vi "RSZVB Set Converter Power Offset.vi"(6 "Port Power Offset (0)":dbl format="%^.3e", 7 "Offset Parameter (1)":i32(ring)=1 items=["Only", "Add Channel Power"], 8 "error in (no error)":errorcluster {"code" format="%.0x"}, 9 "Port (1)":i32=1, 10 "Channel (1)":i32=1, 11 "VISA session":refnum<visa-resource-name>) -> (0 "error out":errorcluster {"code" format="%.0x"}, 3 "dup VISA session":refnum<visa-resource-name>)   [LabVIEW 2011]
doc: "This VI defines a source power or a power offset relative to the channel power (SOURce<Ch>:POWer<Pt>[:LEVel][:IMMediate][:AMPlitude]) for a frequency converter port <Pt>. The command is available for converters with electronic attenuators (R&S ZVA-ZxxxE). An additional Cal Power Offset can be defined via SOURce<Ch>:POWer<Pt>:CORRection:LEVel:OFFSet. \n\n\nNotes:\n\n(1) This command is available for frequency converters with electronic attenuators R&S ZVA-ZxxxE.\n\nRemote-control command(s):\nSOURce<Ch>:POWer<Pt>:CONVerter:OFFSet <numeric_value>, ONLY | CPADd"
uses:
  _utility/RSZVB Global Data.vi
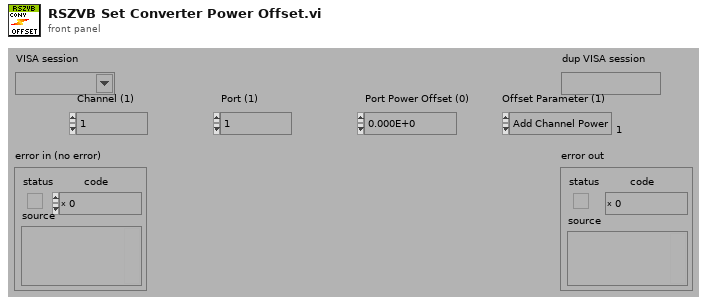
[diagram p1: front panel]
types:
  T1 = cluster{"Error Checking (T: On)":bool, "Installed Options":string[], "Data Valid?":bool, "Ports":i32, "Model":string[], "Option Checking (T: On)":bool}[]
  T2 = cluster{"Error Checking (T: On)":bool, "Installed Options":string[], "Data Valid?":bool, "Ports":i32, "Model":string[], "Option Checking (T: On)":bool}
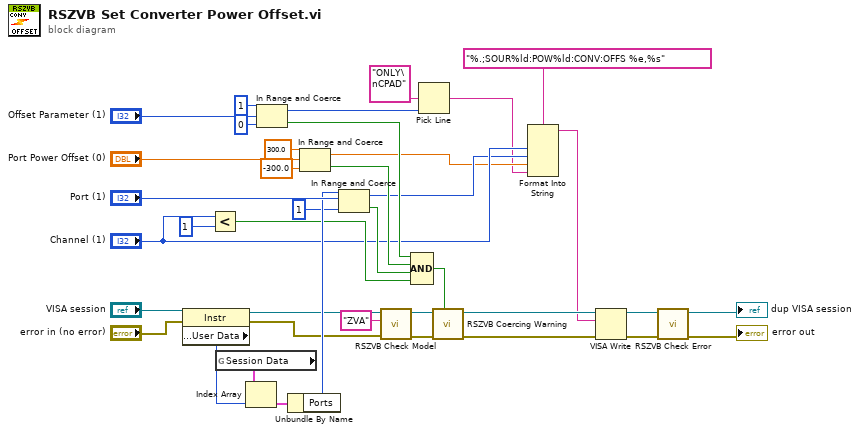
[diagram p0: block diagram]
diagram:
  n1 = property class="Instr"(reference="VISA session", error in="error in (no error)") -> (reference out=w1:refnum<visa-resource-name>, error out=w2:errorcluster, "General Settings:User Data"=w37:u32)
  n2 = Less?(x="Channel (1)", y=1) -> (x < y?=w21:bool)
  n3 = global read "RSZVB Global Data.vi" "Session Data"() -> (w38:T1)
  n4 = Index Array(array=w38, index=w37) -> (element=w39:T2)
  n5 = In Range and Coerce(upper limit=1, x="Offset Parameter (1)", lower limit=0) -> (coerced(x)=w19:i32, In Range?=w24:bool)
  n6 = Unbundle By Name(w39) -> ("Ports"=w33:i32)
  n7 = In Range and Coerce(upper limit=300.0, x="Port Power Offset (0)", lower limit=-300.0) -> (coerced(x)=w14:dbl, In Range?=w23:bool)
  n8 = In Range and Coerce(upper limit=w33, x="Port (1)", lower limit=1) -> (coerced(x)=w15:i32, In Range?=w22:bool)
  n9 = call "RSZVB Check Model.vi"("error in (no error)"=w2, "Model"="ZVA", "VISA session"=w1) -> ("error out"=w4:errorcluster, "dup VISA session"=w3:refnum<visa-resource-name>)  [unwired: 7 in]
  n10 = Compound Arithmetic op=AND(w24, w23, w22, w21) -> (w20:bool)
  n11 = Pick Line(multi-line string="ONLY\nCPAD", line index=w19) -> (output string=w13:string)  [unwired: 1 in]
  n12 = call "RSZVB Coercing Warning.vi"("In Range?"=w20, "error in (no error)"=w4, "VISA session"=w3) -> ("error out"=w11:errorcluster, "dup VISA session"=w12:refnum<visa-resource-name>)  [unwired: 7 in]
  n13 = Format Into String(format string="%.;SOUR%ld:POW%ld:CONV:OFFS %e,%s", "Channel (1)", w15, w14, w13) -> (resulting string=w10:string)  [unwired: 2 in, 1 out]
  n14 = VISA Write(VISA resource name=w12, write buffer=w10, error in (no error)=w11) -> (VISA resource name out=w9:refnum<visa-resource-name>, error out=w8:errorcluster)  [unwired: 1 out]
  n15 = call "RSZVB Check Error.vi"("error in (no error)"=w8, "VISA session"=w9) -> ("error out"=→"error out":errorcluster, "dup VISA session"=→"dup VISA session":refnum<visa-resource-name>)  [unwired: 8 in]
